vi "Main Page.vi"(8 "error in (no error)":errorcluster, 11 "Node Ptr":T2 format="%.0x") -> (0 "error out":errorcluster)   [LabVIEW 2020, in "AIM ARINC 664 System Explorer.lvlib" / "Implementation.lvlib"]
uses:
  Implementation.lvlib
  <vilib>/NI VeriStand/Custom Device API/Custom Device Item Ref.ctl
  <vilib>/NI VeriStand/Custom Device API/Get Item Property (I32).vi
  <vilib>/NI VeriStand/Custom Device API/Custom Device API.lvlib
  Scripting/AIM ARINC 664 Scripting.lvlib
panel:
  in  "SHDocVw.IWebBrowser":refnum<k7>(container)
  in  "Tab Control":enum32{"General", "Interface"}(tab)
  in  "Decimation":i32=1 min=1
  in  "Board ID Number":i32 caption="Board ID" min=0
  in  "initialization method":enum16{"Board Number", "Serial Number"}(ring) caption="Initialization Method"
  out "Ports Speed":T1(ring)
  in  "Inline Tx Generic":bool
  in  "Inline Tx UDP":bool
  in  "Inline Rx UDP":bool
  in  "Outgoing Frame Rate":dbl caption="Outgoing frame processing rate [Hz]" min=0.0
  in  "Incoming Frame Rate":dbl caption="Incoming frame processing rate [Hz]" min=0.0
  in  "Inline Rx Execution":bool caption="Inline Rx Monitor  Execution"
  out "Version":string
  in  "General Header":cluster{"Section Name":string}={"Section Name"="AIM ARINC 664 - Main"}
  in  "Description":string
  in  "Name":string
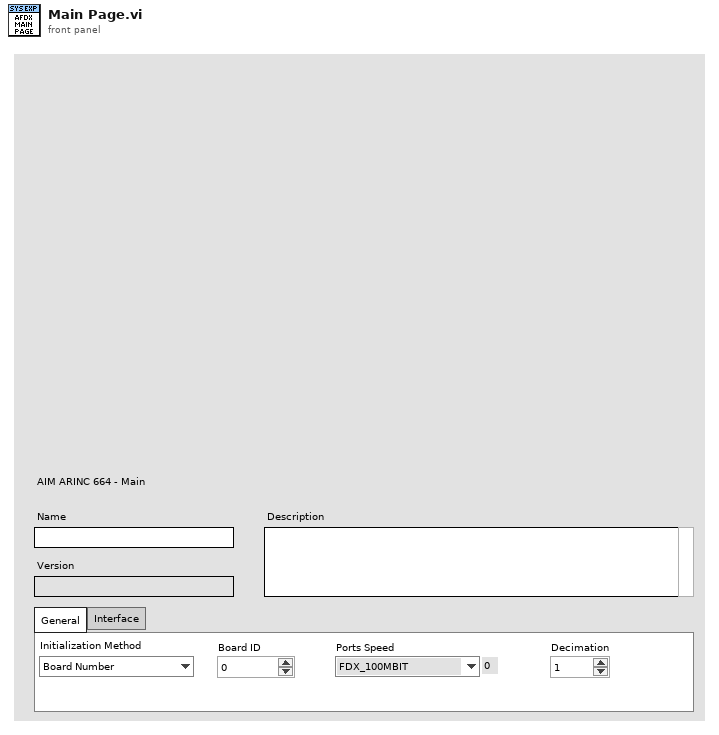
[diagram p1: front panel]
types:
  T1 = enum16{"FDX_100MBIT", "FDX_10MBIT", "FDX_AUTO_100MBIT", "FDX_AUTO_10MBIT", "FDX_AUTO_ERROR", "FDX_1000MBIT"}
  T2 = typedef "Custom Device API.lvlib/Custom Device Item Ref.ctl" = u64
  T3 = typedef "Custom Device API.lvlib/Custom Device Item Info.ctl" = cluster{"Name":string, "Is Channel":bool, "GUID":string, "Is Waveform":bool}
  T4 = typedef "Custom Device API.lvlib/Custom Device Commands.ctl" = enum16{"Default", "Item renamed", "Shutdown", "Dynamic button pressed"}
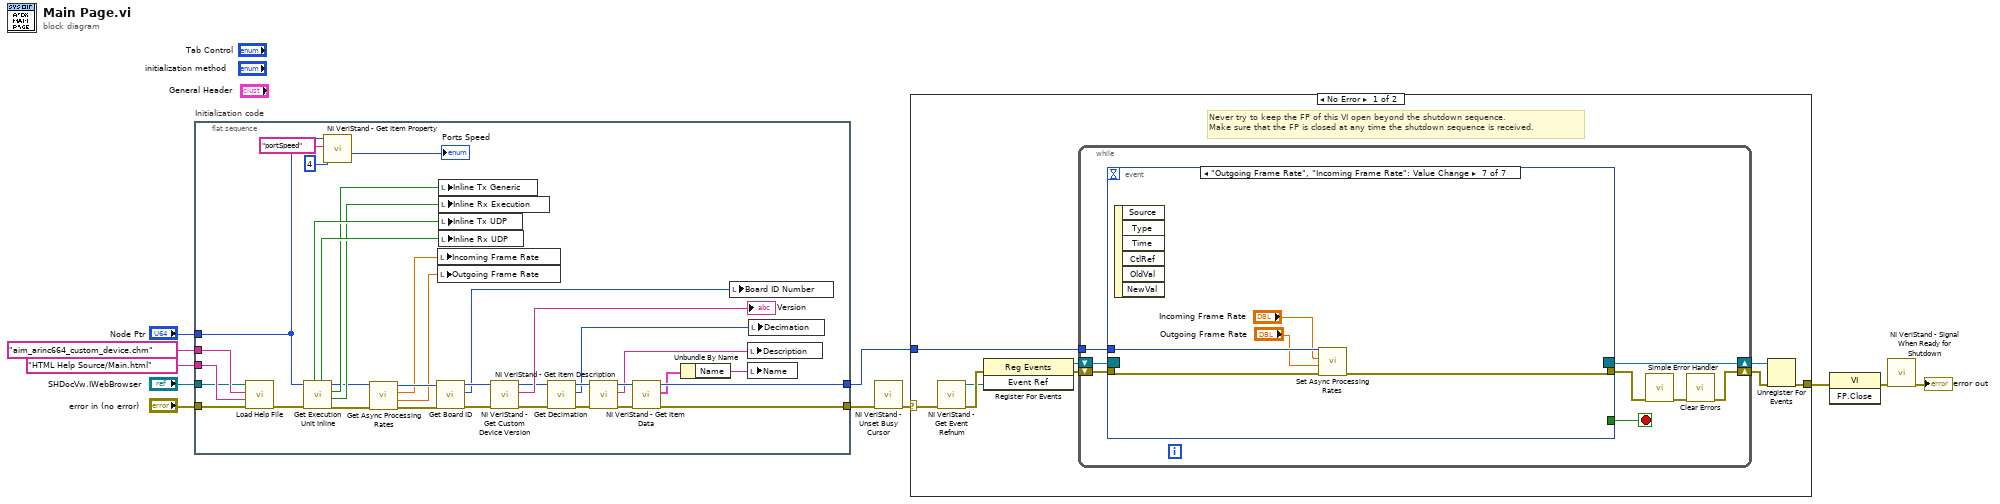
[diagram p0: block diagram]
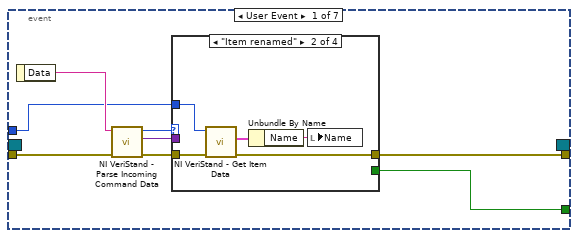
[diagram p2: hidden frame]
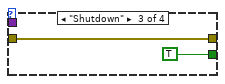
[diagram p4: hidden frame]
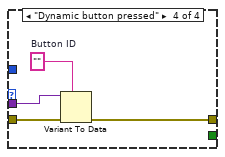
[diagram p5: hidden frame]
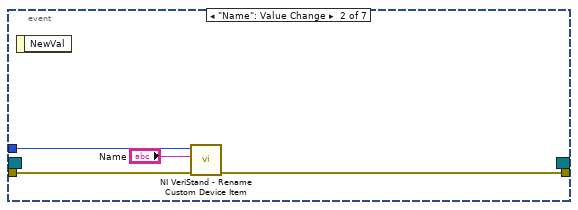
[diagram p6: hidden frame]
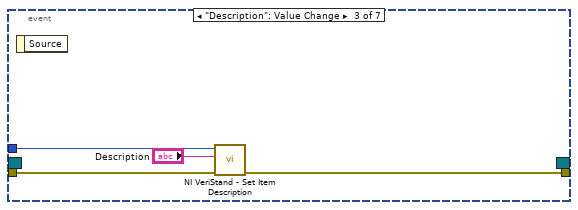
[diagram p7: hidden frame]
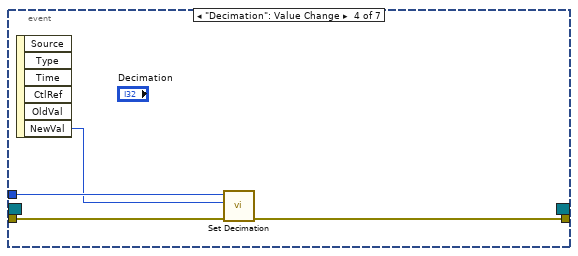
[diagram p8: hidden frame]
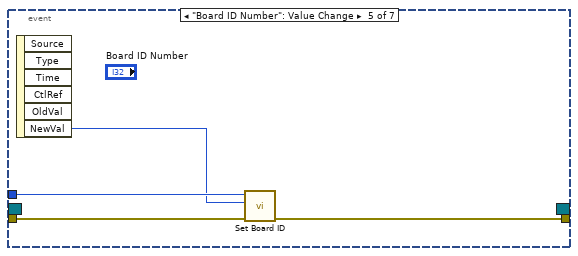
[diagram p9: hidden frame]
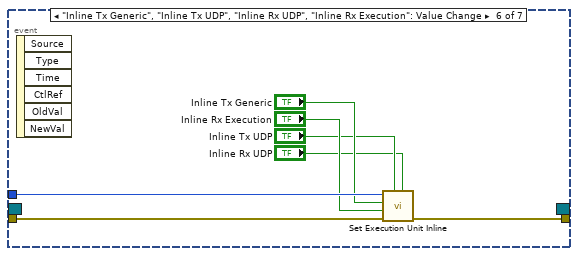
[diagram p10: hidden frame]
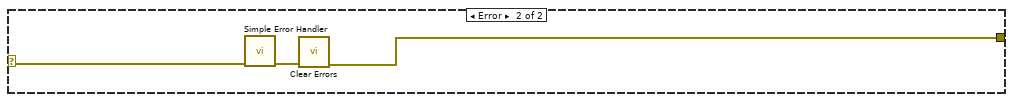
[diagram p11: hidden frame]
diagram:
  n1 = flat-sequence "Initialization code" {
    tunnel: "error in (no error)" -> [w38]
    tunnel: "Node Ptr" -> [w23]
    tunnel: [w42] -> w7
    tunnel: [w46] -> w4
    tunnel: "SHDocVw.IWebBrowser" -> [w35]
    tunnel: "HTML Help Source/Main.html" ("HTML File") -> [w36]
    tunnel: "aim_arinc664_custom_device.chm" ("CD_CHM_FileName") -> [w37]
    frame #0 {
      n2 = call "Load Help File.vi"("error in (no error)"=w38, "HTML File to Load"=w36, "Main CHM File"=w37, "Browser"=w35) -> ("error out"=w22:errorcluster)  [unwired: 6 in, 1 out]
      n3 = call "Get Execution Unit Inline.vi"("error in"=w22, "custom device ref"=w23) -> ("error out"=w16:errorcluster, "Inline Rx Execution"=w18:bool, "Inline Tx Generic"=w19:bool, "custom device ref out"=w17:T2, "Inline Rx UDP"=w20:bool, "Inline Tx UDP"=w21:bool)  [unwired: 4 in]
      n4 = call-poly <vilib>:"NI VeriStand - Get Item Property.vi"("Default Value"=4, "Property Name"="portSpeed", "Item Ref in"=w23) -> ("Value"=→"Ports Speed":i32)  [unwired: 5 in, 3 out]
      n5 = call "Get Async Processing Rates.vi"("error in"=w16, "custom device ref"=w17) -> ("error out"=w15:errorcluster, "Outgoing Frame Rate"=w12:dbl, "Incoming Frame Rate"=w13:dbl, "custom device ref out"=w14:T2)  [unwired: 6 in]
      n6 = call "Get Board ID.vi"("error in"=w15, "custom device ref"=w14) -> ("error out"=w29:errorcluster, "Board ID"=w27:i32, "custom device ref out"=w28:T2)  [unwired: 7 in]
      n7 = local write "Incoming Frame Rate"(w13) -> ()
      n8 = local write "Outgoing Frame Rate"(w12) -> ()
      n9 = local write "Inline Tx Generic"(w19) -> ()
      n10 = local write "Inline Rx Execution"(w18) -> ()
      n11 = local write "Inline Tx UDP"(w21) -> ()
      n12 = local write "Inline Rx UDP"(w20) -> ()
      n13 = call <vilib>:"NI VeriStand - Get Custom Device Version.vi"("error in (no error)"=w29, "Device Ref in"=w28) -> ("error out"=w32:errorcluster, "Value"=→"Version":string, "Device Ref out"=w34:T2)  [unwired: 7 in]
      n14 = call "Get Decimation.vi"("error in"=w32, "custom device ref"=w34) -> ("error out"=w31:errorcluster, "decimation"=w30:i32, "custom device ref out"=w33:T2)  [unwired: 7 in]
      n15 = call <vilib>:"NI VeriStand - Get Item Description.vi"("error in (no error)"=w31, "Item Ref in"=w33) -> ("error out"=w44:errorcluster, "Description"=w39:string, "Item Ref out"=w45:T2)  [unwired: 7 out]
      n16 = call <vilib>:"NI VeriStand - Get Item Data.vi"("error in (no error)"=w44, "Item Ref in"=w45) -> ("error out"=w42:errorcluster, "Item Info"=w43:T3, "Item Ref out"=w46:T2)  [unwired: 7 out]
      n17 = Unbundle By Name(w43) -> ("Name"=w40:string)
      n18 = local write "Board ID Number"(w27) -> ()
      n19 = local write "Description"(w39) -> ()
      n20 = local write "Name"(w40) -> ()
      n21 = local write "Decimation"(w30) -> ()
    }
  }
  n22 = call <vilib>:"NI VeriStand - Unset Busy Cursor.vi"("error in (no error)"=w7) -> ("error out"=w6:errorcluster)  [unwired: 10 out]
  n23 = case shown="No Error" w6 {
    selector: w6 -> [w47 w114]
    tunnel: [w52 w112] -> w11
    tunnel: w4 -> [w48 _]
    frame No Error {
      # "Never try to keep the FP of this VI open beyond the shutdown sequence.\nMake sure that the FP is closed at any time the shutdown sequence is received."
      n24 = call <vilib>:"NI VeriStand - Get Event Refnum.vi"("error in (no error)"=w47) -> ("error out"=w55:errorcluster, "Event Ref"=w51:refnum<user-event>)  [unwired: 9 out]
      n25 = register-events(error in=w55, w51) -> (reference out=w49:refnum<event-registration>, error out=w50:errorcluster)  [unwired: 1 in]
      n26 = while {
        tunnel: w48 -> [w59]
        shift-right: [w56] -> w53
        shift-left: w50 -> [w62]
        shift-right: [w63] -> w54
        shift-left: w49 -> [w61]
        stop <- w60 stop-if-true
        n27 = event shown="[6] \"Outgoing Frame Rate\", \"Incoming Frame Rate\": Value Change" {
          selector: w61 -> [_ _ _ _ _ _ _]
          dyn-events: [_ _ _ _ _ _ _] -> w63
          timeout: _ -> [_ _ _ _ _ _ _]
          tunnel: w62 -> [w71 w87 w90 w95 w99 w106 w110]
          tunnel: [w67 _ _ _ _ _ _] -> w60
          tunnel: [w66 w86 w89 w92 w98 w105 w107] -> w58
          tunnel: w59 -> [w65 w85 w91 w94 w97 w104 w111]
          event User Event {
            n28 = event-data() -> ("Data"=w70:string)  [unwired: 1 out]
            n29 = call <vilib>:"NI VeriStand - Parse Incoming Command Data.vi"("error in (no error)"=w71, "Incoming data"=w70) -> ("error out"=w69:errorcluster, "Outgoing data"=w64:variant, "Action"=w68:T4)  [unwired: 7 out]
            n30 = case shown="\"Item renamed\"" w68 {
              tunnel: w69 -> [w72 w77 w78 w83]
              tunnel: [_ _ TRUE _] -> w67
              tunnel: [w72 w74 w78 w80] -> w66
              tunnel: w65 -> [_ w76 _ _]
              tunnel: w64 -> [_ _ _ w82]
              frame "Default", Default {
              }
              frame "Item renamed" {
                n31 = call <vilib>:"NI VeriStand - Get Item Data.vi"("error in (no error)"=w77, "Item Ref in"=w76) -> ("error out"=w74:errorcluster, "Item Info"=w75:T3)  [unwired: 8 out]
                n32 = Unbundle By Name(w75) -> ("Name"=w73:string)
                n33 = local write "Name"(w73) -> ()
              }
              frame "Shutdown" {
              }
              frame "Dynamic button pressed" {
                w81 = ""  # Button ID
                n34 = Variant To Data(error in=w83, type=w81, Variant=w82) -> (error out=w80:errorcluster)  [unwired: 1 out]
              }
            }
          }
          event "Name": Value Change {
            n35 = event-data() -> ()  [unwired: 2 out]
            n36 = call <vilib>:"NI VeriStand - Rename Custom Device Item.vi"("error in (no error)"=w87, "New Name"="Name", "Item Ref in"=w85) -> ("error out"=w86:errorcluster)  [unwired: 1 in, 7 out]
          }
          event "Description": Value Change {
            n37 = event-data() -> ()  [unwired: 2 out]
            n38 = call <vilib>:"NI VeriStand - Set Item Description.vi"("error in (no error)"=w90, "Description"="Description", "Item Ref in"=w91) -> ("error out"=w89:errorcluster)  [unwired: 8 out]
          }
          event "Decimation": Value Change {
            n39 = event-data() -> ("NewVal"=w93:i32)  [unwired: 6 out]
            n40 = call "Set Decimation.vi"("error in"=w95, "decimation"=w93, "custom device ref"=w94) -> ("error out"=w92:errorcluster)  [unwired: 7 in, 1 out]
          }
          event "Board ID Number": Value Change {
            n41 = event-data() -> ("NewVal"=w96:i32)  [unwired: 6 out]
            n42 = call "Set Board ID.vi"("error in"=w99, "Board ID"=w96, "custom device ref"=w97) -> ("error out"=w98:errorcluster)  [unwired: 7 in, 1 out]
          }
          event "Inline Tx Generic", "Inline Tx UDP", "Inline Rx UDP", "Inline Rx Execution": Value Change {
            n43 = event-data() -> ()  [unwired: 7 out]
            n44 = call "Set Execution Unit Inline.vi"("Inline Rx UDP"="Inline Rx UDP", "Inline Tx UDP"="Inline Tx UDP", "error in"=w106, "Inline Inline Rx Monitor"="Inline Rx Execution", "Inline Tx Generic Execution"="Inline Tx Generic", "custom device ref"=w104) -> ("error out"=w105:errorcluster)  [unwired: 4 in, 1 out]
          }
          event "Outgoing Frame Rate", "Incoming Frame Rate": Value Change {
            n45 = event-data() -> ()  [unwired: 7 out]
            n46 = call "Set Async Processing Rates.vi"("error in"=w110, "Outgoing Frame Rate"="Outgoing Frame Rate", "Incoming Frame Rate"="Incoming Frame Rate", "custom device ref"=w111) -> ("error out"=w107:errorcluster)  [unwired: 6 in, 1 out]
          }
        }
        n47 = call <vilib>:"Simple Error Handler.vi"("error in (no error)"=w58) -> ("error out"=w57:errorcluster)  [unwired: 1 in, 7 out]
        n48 = call <vilib>:"Clear Errors.vi"("error in (no error)"=w57) -> ("error out"=w56:errorcluster)  [unwired: 1 in, 5 out]
      }
      n49 = Unregister For Events(event registration refnum=w54, error in=w53) -> (error out=w52:errorcluster)
    }
    frame Error {
      n50 = call <vilib>:"Simple Error Handler.vi"("error in (no error)"=w114) -> ("error out"=w113:errorcluster)  [unwired: 1 in, 7 out]
      n51 = call <vilib>:"Clear Errors.vi"("error in (no error)"=w113) -> ("error out"=w112:errorcluster)  [unwired: 1 in, 5 out]
    }
  }
  n52 = invoke class="VI" method="FP.Close"(error in=w11) -> (error out=w10:errorcluster)  [unwired: 2 in, 2 out]
  n53 = call <vilib>:"NI VeriStand - Signal When Ready for Shutdown.vi"("error in (no error)"=w10) -> ("error out"=→"error out":errorcluster)  [unwired: 10 out]
